vi "Averaged Cross Spectrum (Mag-Phase).vi"(0 "scaled signal X [EUx]":dbl[](array[numeric]) format="%.2f", 1 "scaled signal Y [EUy]":dbl[](array[numeric]) format="%.2f", 2 "sampling frequency [Hz]":dbl=10000.0 format="%.2f", 3 "view":T5, 4 "channel X info":T2={"sensor sensitivity [mV/EU]"=1000.0, "engineering units"=1, "dB reference [EU]"=1.0, "custom label"="EU", "weighting filter"=0, "pregain [dB]"=0.0} {"pregain [dB]" format="%.2f"; "weighting filter" items=["Linear", "A-weighting", "B-weighting", "C-weighting", "ITU-R 468-4", "Dolby", "CCITT", "C-message"]; "dB reference [EU]" format="%^.1e"; "engineering units" items=["custom..."=0, "V"=1, "A"=21, "Pa"=2, "N"=20, "g"=3, "m/s^2"=4, "m/s"=5, "m"=6, "mm/s"=12, "mm"=13, "microns/s"=14, "microns"=15, "in/s^2"=7, "in/s"=8, "in"=9, "mils/s"=10, "mils"=11, "rad/s^2"=16, "rad/s"=17, "rad"=18, "strain"=19]; "sensor sensitivity [mV/EU]" format="%.2f"}, 5 "channel Y info":T2={"sensor sensitivity [mV/EU]"=1000.0, "engineering units"=1, "dB reference [EU]"=1.0, "custom label"="EU", "weighting filter"=0, "pregain [dB]"=0.0} {"pregain [dB]" format="%.2f"; "weighting filter" items=["Linear", "A-weighting", "B-weighting", "C-weighting", "ITU-R 468-4", "Dolby", "CCITT", "C-message"]; "dB reference [EU]" format="%^.1e"; "engineering units" items=["custom..."=0, "V"=1, "A"=21, "Pa"=2, "N"=20, "g"=3, "m/s^2"=4, "m/s"=5, "m"=6, "mm/s"=12, "mm"=13, "microns/s"=14, "microns"=15, "in/s^2"=7, "in/s"=8, "in"=9, "mils/s"=10, "mils"=11, "rad/s^2"=16, "rad/s"=17, "rad"=18, "strain"=19]; "sensor sensitivity [mV/EU]" format="%.2f"}, 6 "window":T7=1 items=["None"=0, "Hanning"=1, "Hamming"=2, "Blackman-Harris"=3, "Exact Blackman"=4, "Blackman"=5, "Flat Top"=6, "4 Term B-Harris "=7, "7 Term B-Harris"=8, "Low Sidelobe"=9, "Force - Exponential"=10, "Blackman Nuttall"=11, "Triangle"=30, "Bartlett-Hanning"=31, "Bohman"=32, "Parzen"=33, "Welch"=34, "Kaiser"=60, "Dolph-Chebyshev"=61, "Gaussian"=62], 7 "reset averaging (T)":bool=TRUE, 8 "force/exp settings":T6={"force window [%]"=50.0, "exponential window [%]"=10.0} {"exponential window [%]" min=0.0 max=100.0 format="%.2f"; "force window [%]" min=0.0 max=100.0 format="%.2f"}, 9 "averaging parameters":T1={"averaging mode"=enum."RMS averaging", "weighting mode"=enum."Linear", "number of averages"=10} {"number of averages" min=1}) -> (12 "df [Hz]":dbl format="%.2f", 13 "window constants":cluster{"eq noise BW":dbl, "coherent gain":dbl} {"coherent gain" format="%.2f"; "eq noise BW" format="%.2f"}, 14 "magnitude [EUx EUy rms]":dbl[](array[numeric]) format="%.2f", 15 "unit label (magnitude)":string, 16 "phase":dbl[](array[numeric]) format="%.2f", 17 "unit label (phase)":string, 18 "averages completed":dbl format="%.2f", 19 "error out":errorcluster)   [LabVIEW 2017]
doc: "Computes the averaged cross power spectrum of the input signals. Typically, X signal is the stimulus, and Y signal is the response of the system. Results are returned as magnitude and phase.\nEach block of data corresponds to a single FFT block and has to be passed individually to this VI. The first time this VI is called, reset averaging must be TRUE (default value) to start a new averaging process. For subsequent calls, reset averaging must be FALSE to continue the averaging process. Averages completed returns the number of averages completed so far.\nAveraging parameters specifies how the averaging is performed. This includes the averaging mode (no averaging, vector averaging, or RMS averaging), the weighting mode (linear or exponential) and the number of averages (used only if the weighting mode is exponential).\nThe view cluster allows you to display magnitude results in decibels, and the phase results unwrapped or not, in radians or degrees."
uses:
  <vilib>/addons/_NISVFA/_Shared subVIs/Controls/svc_Window [Dual FFT].ctl
  <vilib>/addons/Sound and Vibration/compatibility/Controls/svl_Channel Info.ctl
  <vilib>/addons/Sound and Vibration/compatibility/Controls/svl_Engineering Units Text Ring.ctl
  <vilib>/addons/Sound and Vibration/compatibility/Controls/svl_Weighting Filter Text Ring.ctl
  <vilib>/Analysis/4window.llb/Force Window (DBL).vi
  <vilib>/Analysis/4window.llb/Exponential Window (DBL).vi
  <vilib>/Analysis/2dsp.llb/Cross Power (DBL).vi
  <vilib>/Analysis/2dsp.llb/Real FFT.vi
  <vilib>/Analysis/0measdsp.llb/Scaled Time Domain Window (DBL).vi
  <vilib>/Analysis/NI_AALPro.lvlib
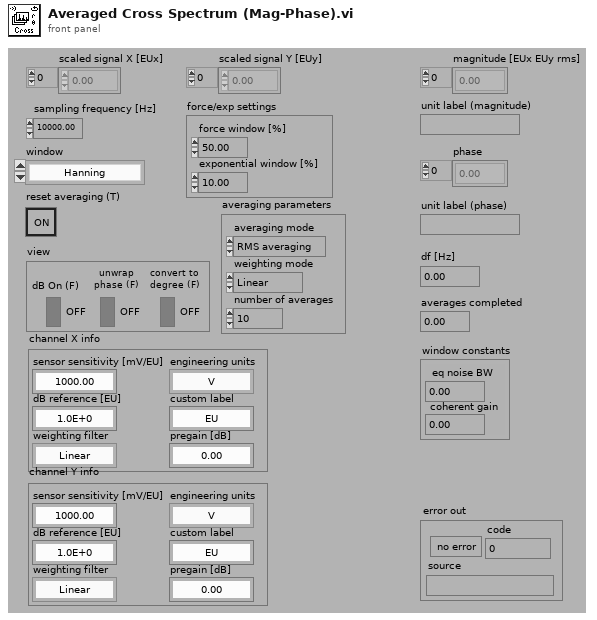
[diagram p1: front panel]
types:
  T1 = cluster{"averaging mode":enum16{"No averaging", "Vector averaging", "RMS averaging"}, "weighting mode":enum16{"Linear", "Exponential"}, "number of averages":u32}
  T2 = typedef "svl_Channel Info.ctl" = cluster{"sensor sensitivity [mV/EU]":dbl, "engineering units":T3, "dB reference [EU]":dbl, "custom label":string, "weighting filter":T4, "pregain [dB]":dbl}
  T3 = typedef "svl_Engineering Units Text Ring.ctl" = u16
  T4 = typedef "svl_Weighting Filter Text Ring.ctl" = u16
  T5 = cluster{"dB On (F)":bool, "unwrap phase (F)":bool, "convert to degree (F)":bool}
  T6 = cluster{"force window [%]":dbl, "exponential window [%]":dbl}
  T7 = typedef "svc_Window [Dual FFT].ctl" = u32
  T8 = enum16{"No averaging", "Vector averaging", "RMS averaging"}
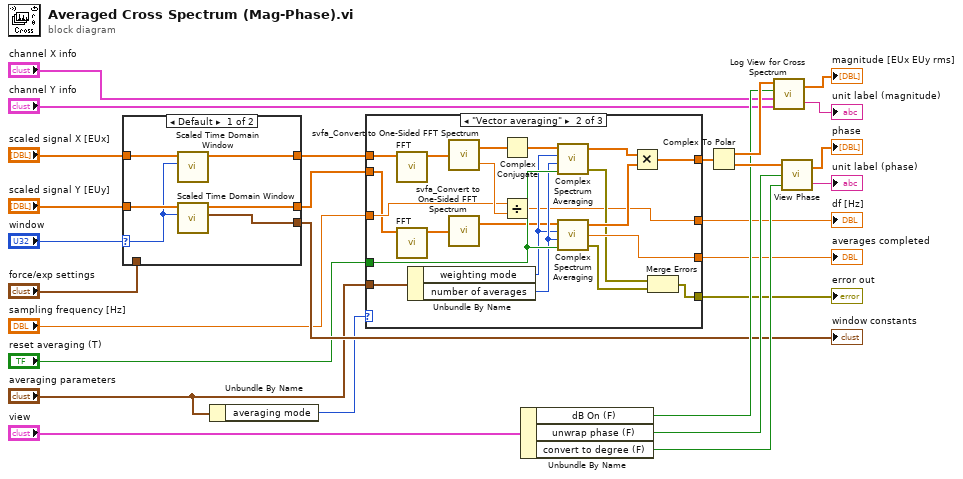
[diagram p0: block diagram]
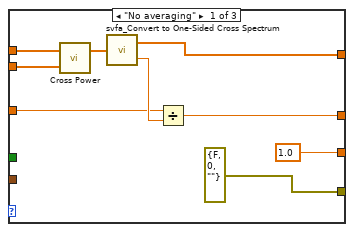
[diagram p2: hidden frame]
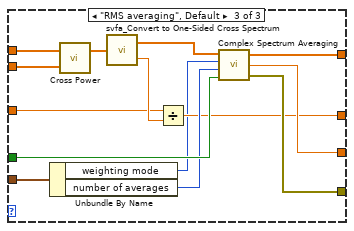
[diagram p3: hidden frame]
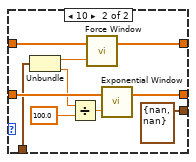
[diagram p4: hidden frame]
diagram:
  n1 = case shown="Default" "window" {
    selector: "window" -> [w28 _]
    tunnel: "scaled signal X [EUx]" -> [w33 w43]
    tunnel: "scaled signal Y [EUy]" -> [w32 w42]
    tunnel: "force/exp settings" -> [_ w38]
    tunnel: [w31 w40] -> w12
    tunnel: [w30 w39] -> w11
    tunnel: [w29 cluster{"eq noise BW":dbl, "coherent gain":dbl} {"eq noise BW"=nan, "coherent gain"=nan} ("window constants")] -> w13
    frame Default {
      n2 = call-poly <vilib>:"Scaled Time Domain Window.vi"("window"=w28, "X"=w33) -> ("Windowed X"=w31:dbl[])  [unwired: 7 in, 2 out]
      n3 = call-poly <vilib>:"Scaled Time Domain Window.vi"("window"=w28, "X"=w32) -> ("window properties"=w29:cluster{"eq noise BW":dbl, "coherent gain":dbl}, "Windowed X"=w30:dbl[])  [unwired: 7 in, 1 out]
    }
    frame 10 {
      n4 = Unbundle(w38) -> ("force window [%]"=w37:dbl, "exponential window [%]"=w36:dbl)
      n5 = Divide(x=w36, y=100.0 ("x")) -> (x/y=w41:dbl)
      n6 = call-poly <vilib>:"Force Window.vi"("duty cycle(%)"=w37, "X"=w43) -> ("Windowed X"=w40:dbl[])  [unwired: 1 out]
      n7 = call-poly <vilib>:"Exponential Window.vi"("final value"=w41, "X"=w42) -> ("Windowed X"=w39:dbl[])  [unwired: 1 out]
    }
  }
  "window constants" <- w13
  n8 = Unbundle By Name("averaging parameters") -> ("averaging mode"=w7:T8)
  n9 = case shown="\"Vector averaging\"" w7 {
    tunnel: w12 -> [w48 w59 w79]
    tunnel: w11 -> [w47 w55 w78]
    tunnel: "sampling frequency [Hz]" -> [w46 w57 w77]
    tunnel: [w44 w56 w75] -> w4
    tunnel: [w45 w67 w84] -> w6
    tunnel: "reset averaging (T)" -> [_ w71 w87]
    tunnel: "averaging parameters" -> [_ w72 w86]
    tunnel: [1.0 ("averages completed") w69 w83] -> w5
    tunnel: [errorcluster {"status"=FALSE, "code"=0, "source"=""} ("error out") w65 w82] -> w1
    frame "No averaging" {
      n10 = call-poly <vilib>:"Cross Power.vi"("Y"=w47, "X"=w48) -> ("Sxy"=w49:cdb[])  [unwired: 1 out]
      n11 = call <vilib>:"svfa_Convert to One-Sided Cross Spectrum.vi"("two-sided cross spectrum"=w49) -> ("one-sided cross spectrum"=w45:cdb[], "block size"=w50:dbl)
      n12 = Divide(x=w46, y=w50) -> (x/y=w44:dbl)
    }
    frame "Vector averaging" {
      n13 = call-poly <vilib>:"FFT.vi"("X"=w59) -> ("FFT {X}"=w61:cdb[])  [unwired: 9 in, 1 out]
      n14 = call-poly <vilib>:"FFT.vi"("X"=w55) -> ("FFT {X}"=w54:cdb[])  [unwired: 9 in, 1 out]
      n15 = Unbundle By Name(w72) -> ("weighting mode"=w64:enum16{"Linear", "Exponential"}, "number of averages"=w70:u32)
      n16 = call <vilib>:"svfa_Convert to One-Sided FFT Spectrum.vi"("two-sided FFT spectrum"=w61) -> ("one-sided FFT spectrum"=w58:cdb[], "block size"=w60:dbl)
      n17 = call <vilib>:"svfa_Convert to One-Sided FFT Spectrum.vi"("two-sided FFT spectrum"=w54) -> ("one-sided FFT spectrum"=w53:cdb[])  [unwired: 1 out]
      n18 = Complex Conjugate(1:w58) -> (0:w73:cdb[])
      n19 = Divide(x=w57, y=w60) -> (x/y=w56:dbl)
      n20 = call <vilib>:"Complex Spectrum Averaging.vi"("reset averaging (T)"=w71, "number of averages"=w70, "weighting mode"=w64, "complex spectrum"=w73) -> ("error out"=w63:errorcluster, "averaged complex spectrum"=w68:cdb[])  [unwired: 1 out]
      n21 = call <vilib>:"Complex Spectrum Averaging.vi"("reset averaging (T)"=w71, "number of averages"=w70, "weighting mode"=w64, "complex spectrum"=w53) -> ("error out"=w62:errorcluster, "averages completed"=w69:dbl, "averaged complex spectrum"=w66:cdb[])
      n22 = Multiply(x=w68, y=w66) -> (x*y=w67:cdb[])
      n23 = Merge Errors(w63, w62) -> (w65:errorcluster)
    }
    frame "RMS averaging", Default {
      n24 = Unbundle By Name(w86) -> ("weighting mode"=w74:enum16{"Linear", "Exponential"}, "number of averages"=w85:u32)
      n25 = call-poly <vilib>:"Cross Power.vi"("Y"=w78, "X"=w79) -> ("Sxy"=w80:cdb[])  [unwired: 1 out]
      n26 = call <vilib>:"svfa_Convert to One-Sided Cross Spectrum.vi"("two-sided cross spectrum"=w80) -> ("one-sided cross spectrum"=w76:cdb[], "block size"=w81:dbl)
      n27 = Divide(x=w77, y=w81) -> (x/y=w75:dbl)
      n28 = call <vilib>:"Complex Spectrum Averaging.vi"("reset averaging (T)"=w87, "number of averages"=w85, "weighting mode"=w74, "complex spectrum"=w76) -> ("error out"=w82:errorcluster, "averages completed"=w83:dbl, "averaged complex spectrum"=w84:cdb[])
    }
  }
  "df [Hz]" <- w4
  "averages completed" <- w5
  "error out" <- w1
  n29 = Unbundle By Name("view") -> ("dB On (F)"=w16:bool, "unwrap phase (F)"=w18:bool, "convert to degree (F)"=w17:bool)
  n30 = Complex To Polar(r * e^(i*theta)=w6) -> (r=w20:dbl[], theta=w23:dbl[])
  n31 = call <vilib>:"Log View for Cross Spectrum.vi"("channel Y info"="channel Y info", "channel X info"="channel X info", "dB On (T)"=w16, "cross spectrum [EUx EUy rms]"=w20) -> ("unit label"=→"unit label (magnitude)":string, "log view cross spectrum [dB EUx EUy]"=→"magnitude [EUx EUy rms]":dbl[])
  n32 = call <vilib>:"View Phase.vi"("convert to degree (F)"=w17, "unwrap phase (F)"=w18, "phase (radian)"=w23) -> ("unit label (phase)"=→"unit label (phase)":string, "scaled phase"=→"phase":dbl[])
